vi "confirm commands.vi"() -> ()   [LabVIEW 2020]
uses:
  <vilib>/Instr/_visa.llb/VISA Configure Serial Port (Instr).vi
panel:
  out "x/y":dbl
  out "Waveform Graph":i32[](graph)
  out "Array":T1(array[cluster])
  out "bytes at port 2":u32
  out "error out":errorcluster
  out "read buffer":string
  in  "respons":i32 format="%x"
  out "command worked":bool
  in  "clear command flag":bool
  in  "comment":string
  out "readback":string
  in  "Command":i32 format="%x"
  out "Response string":string
  out "Respons hex":i32 format="%x"
  in  "Stop":bool
  in  "Write":bool
  out "bytes at port":u32
  out "reading":bool
  out "Command":string="*IDN?"
  in  "Command":i32 format="%x"
  in  "store":bool
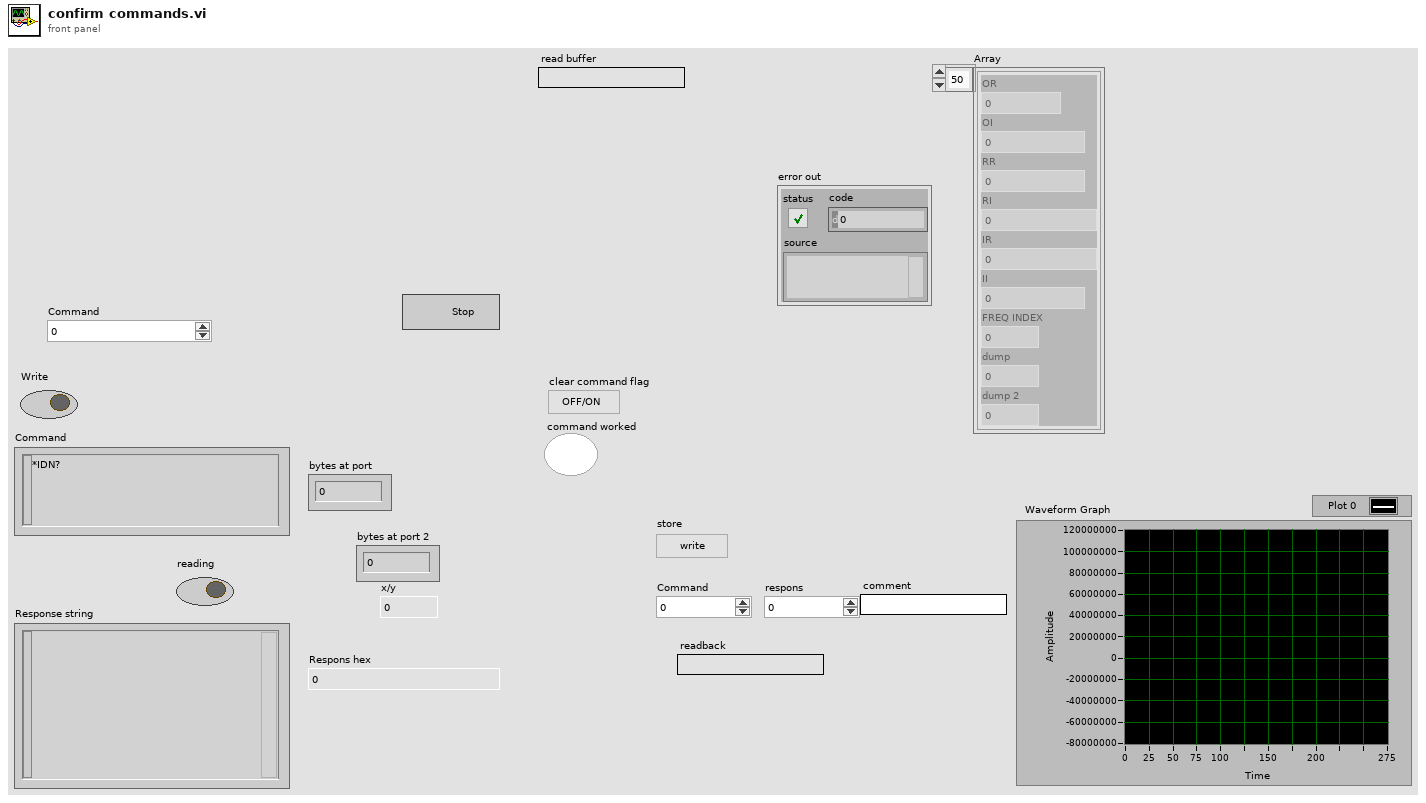
[diagram p1: front panel]
types:
  T1 = cluster{"OR":i32, "OI":i32, "RR":i32, "RI":i32, "IR":i32, "II":i32, "FREQ INDEX":u16, "dump":u16, "dump 2":u32}[]
  T2 = cluster{"baud rate":u32, "data bits":u16, "parity":enum16{"None", "Odd", "Even", "Mark", "Space"}, "stop bits":u16, "flow control":u16}
  T3 = enum16{"open", "replace", "create", "open or create", "replace or create", "replace or create with confirmation"}
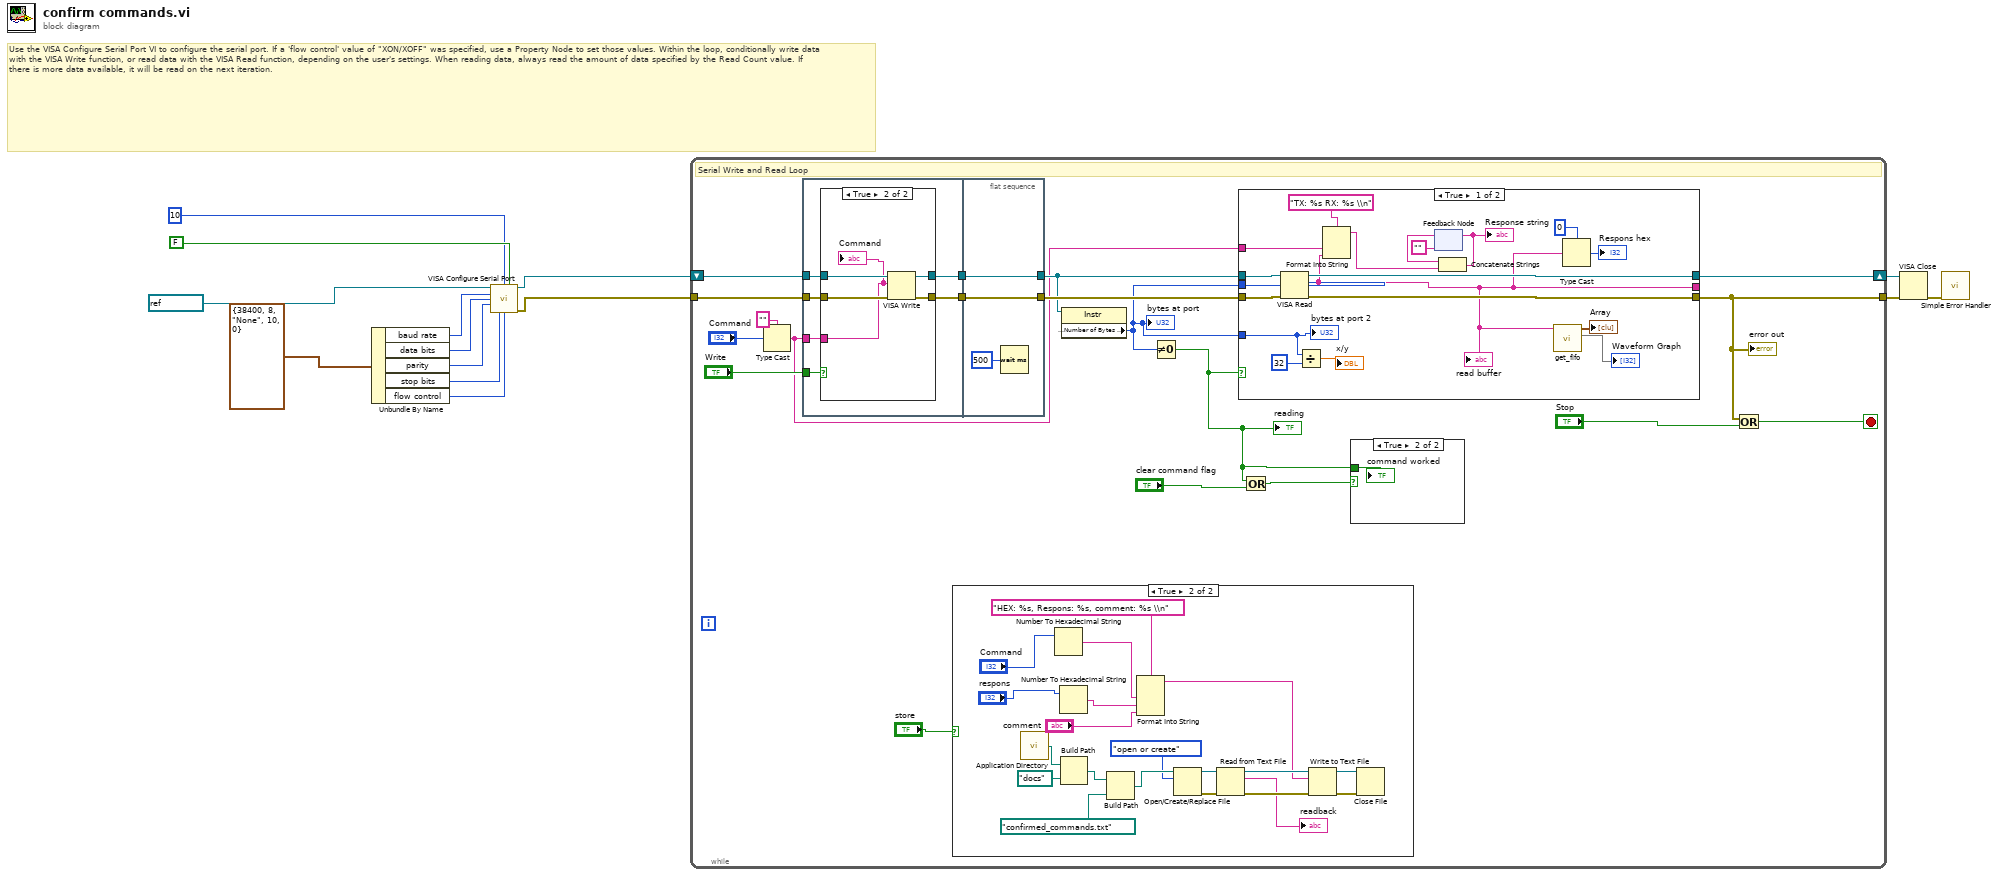
[diagram p0: block diagram]
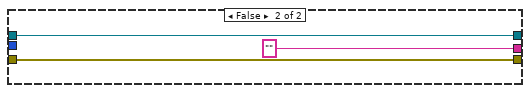
[diagram p5: hidden frame]
diagram:
  # "Use the VISA Configure Serial Port VI to configure the serial port. If a 'flow control' value of \"XON/XOFF\" was specified, use a Property Node to set those values. Within the loop, conditionally write data with the VISA Write function, or read data with the VISA Read function, depending on the user's settings. When reading data, always read the amount of data specified by the Read Count value. If there is more data available, it will be read on the next iteration."
  n1 = Unbundle By Name(T2 {"baud rate"=38400, "data bits"=8, "parity"=enum."None", "stop bits"=10, "flow control"=0} ("Serial Settings")) -> ("baud rate"=w7:u32, "data bits"=w8:u16, "parity"=w9:enum16{"None", "Odd", "Even", "Mark", "Space"}, "stop bits"=w10:u16, "flow control"=w4:u16)
  n2 = call-poly "VISA Configure Serial Port"("VISA resource name"=refnum<visa-resource-name> "COM4", "termination char\n(0xA = '\\n' = LF)"=u8 10 ("Termination Character"), "Enable Termination\nChar (T)"=FALSE ("End Read on Termination Character?"), "baud rate (9600)"=w7, "data bits (8)"=w8, "parity (0:none)"=w9, "stop bits (10: 1 bit)"=w10, "flow control (0:none)"=w4) -> ("VISA resource name out"=w2:refnum<visa-resource-name>, "error out"=w1:errorcluster)  [unwired: 2 in, 4 out]
  n3 = while {
    shift-right: [w33] -> w12
    shift-left: w2 -> [w32]
    tunnel: w1 -> [w31]
    tunnel: [w28] -> w13
    stop <- w29 stop-if-true
    # "Serial Write and Read Loop"
    n4 = Type Cast(type="", x="Command") -> (*(type *) &x=w16:string)
    n5 = flat-sequence {
      tunnel: w32 -> [w60]
      tunnel: w31 -> [w59]
      tunnel: "Write" -> [w56]
      tunnel: w16 -> [w55]
      tunnel: [w58] -> w24
      tunnel: [w57] -> w23
      tunnel: [w69] -> w30
      tunnel: [w70] -> w22
      tunnel: w24 -> [w70]
      tunnel: w23 -> [w69]
      frame #0 {
        n6 = case shown="True" w56 {
          tunnel: w60 -> [w62 w67]
          tunnel: w59 -> [w61 w66]
          tunnel: [w62 w65] -> w58
          tunnel: [w61 w64] -> w57
          tunnel: w55 -> [_ w63]
          frame False {
          }
          frame True {
            n7 = VISA Write(VISA resource name=w67, write buffer=w63, error in (no error)=w66) -> (VISA resource name out=w65:refnum<visa-resource-name>, error out=w64:errorcluster)  [unwired: 1 out]
            "Command" <- w63
          }
        }
      }
      frame #1 {
        n8 = Wait (ms)(milliseconds to wait=u32 500) -> ()  [unwired: 1 out]
      }
    }
    n9 = case shown="True" "store" {
      frame False {
      }
      frame True {
        n10 = call <vilib>:"Application Directory.vi"() -> ("Application Directory"=w48:path)
        n11 = Number To Hexadecimal String(2:"Command") -> (0:w39:string)  [unwired: 1 in]
        n12 = Number To Hexadecimal String(2:"respons") -> (0:w35:string)  [unwired: 1 in]
        n13 = Build Path(base path=w48, name or relative path=path "docs") -> (appended path=w46:path)
        n14 = Build Path(base path=w46, name or relative path=path "confirmed_commands.txt") -> (appended path=w44:path)
        n15 = Format Into String(format string="HEX: %s, Respons: %s, comment: %s \\n", w39, w35, "comment") -> (resulting string=w37:string)  [unwired: 2 in, 1 out]
        n16 = Open/Create/Replace File(file path (use dialog)=w44, operation (0:open)=T3."open or create") -> (refnum out=w54:refnum<file>, error out=w53:errorcluster)  [unwired: 4 in, 1 out]
        n17 = Read from Text File(file (use dialog)=w54, error in=w53) -> (refnum out=w52:refnum<file>, text=→"readback":string, error out=w51:errorcluster)  [unwired: 2 in, 1 out]
        n18 = Write to Text File(file (use dialog)=w52, text=w37, error in=w51) -> (refnum out=w49:refnum<file>, error out=w50:errorcluster)  [unwired: 1 in, 1 out]
        n19 = Close File(refnum=w49, error in=w50) -> ()  [unwired: 2 out]
      }
    }
    n20 = property class="Instr"(reference=w22) -> ("Serial Settings:Number of Bytes at Serial Port"=w15:u32)  [unwired: 1 in, 2 out]
    "bytes at port" <- w15
    n21 = Not Equal To 0?(x=w15) -> (x != 0?=w17:bool)
    "reading" <- w17
    n22 = case shown="True" w17 {
      tunnel: [w87 w92] -> w33
      tunnel: w22 -> [w89 w92]
      tunnel: [w86 w91] -> w28
      tunnel: w30 -> [w88 w91]
      tunnel: w15 -> [w82 _]
      tunnel: [w76 "" ("read buffer")] -> _
      tunnel: w16 -> [w77 _]
      tunnel: w15 -> [w73 _]
      frame True {
        n23 = VISA Read(VISA resource name=w89, byte count=w82, error in (no error)=w88) -> (VISA resource name out=w87:refnum<visa-resource-name>, read buffer=w76:string, error out=w86:errorcluster)  [unwired: 1 out]
        "read buffer" <- w76
        n24 = Divide(x=w73, y=u32 32) -> (x/y=→"x/y":dbl)
        n25 = Format Into String(format string="TX: %s RX: %s \\n", w77, w76) -> (resulting string=w78:string)  [unwired: 2 in, 1 out]
        n26 = feedback #1("") -> (w85:string)
        n27 = Concatenate Strings(w85, w78) -> (w84:string)
        "Response string" <- w84
        n28 = feedback-in #1(w84) -> ()
        n29 = call "get_fifo.vi"("FIFO"=w76) -> (2:→"Waveform Graph", "Array"=→"Array":T1)  [unwired: 8 in, 1 out]
        n30 = Type Cast(type=0 ("Numeric"), x=w76) -> (*(type *) &x=→"Respons hex":i32)
        "bytes at port 2" <- w73
      }
      frame False {
      }
    }
    "error out" <- w28
    n31 = Or(x=w17, y="clear command flag") -> (x .or. y?=w19:bool)
    n32 = case shown="True" w19 {
      tunnel: w17 -> [_ w34]
      frame False {
      }
      frame True {
        "command worked" <- w34
      }
    }
    n33 = Or(x=w28, y="Stop") -> (x .or. y?=w29:bool)
  }
  n34 = VISA Close(VISA resource name=w12, error in (no error)=w13) -> (error out=w14:errorcluster)
  n35 = call <vilib>:"Simple Error Handler.vi"("error in (no error)"=w14) -> ()  [unwired: 1 in, 8 out]
